vi "Create_Image_From_Pixmap_ARGB.vi"(8 "error in (no error)":errorcluster, 10 "Pixmap Image data":T1) -> (0 "error out":errorcluster, 3 "New ARGB Image":refnum<data-value>)   [LabVIEW 2020, in "g_ar_toolkit.lvlib"]
uses:
  g_ar_toolkit.lvlib
  <vilib>/picture/picture.llb/imagedata.ctl
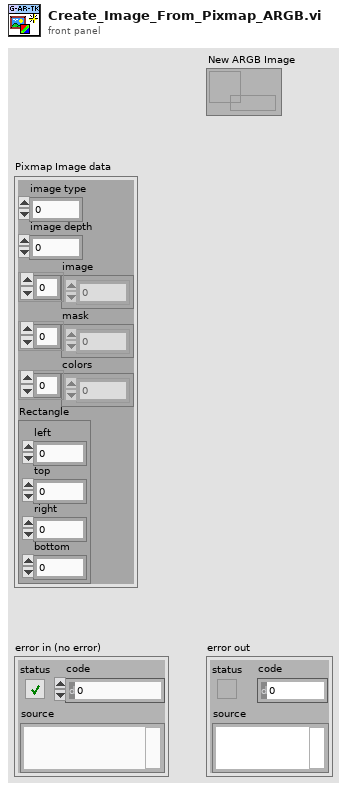
[diagram p1: front panel]
types:
  T1 = typedef "imagedata.ctl" = cluster{"image type":i32, "image depth":i32, "image":u8[], "mask":u8[], "colors":u32[], "Rectangle":cluster{"left":i16, "top":i16, "right":i16, "bottom":i16}}
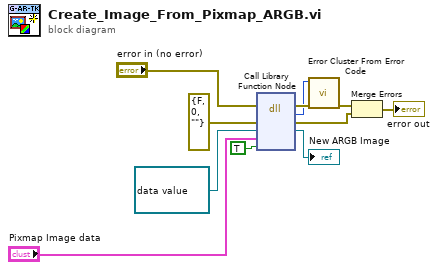
[diagram p0: block diagram]
diagram:
  n1 = dll-call lib="C:/serenial/libraries/g-augmented-reality-toolkit/LabVIEW/g_ar_toolkit/g_ar_toolkit.*.*" fn="Call Library Function Node"(error in="error in (no error)", "error_cluster"=errorcluster {"status"=FALSE, "code"=0, "source"=""} ("error constant"), "EDVR"=refnum<data-value> refnum, "ImageSize"="Pixmap Image data", "is_bgra"=TRUE) -> (error out=w7:errorcluster, "MgErr"=w6:i32, "error_cluster"=w1:errorcluster, "EDVR"=→"New ARGB Image":refnum<data-value>)  [unwired: 4 in, 1 out]
  n2 = call <vilib>:"Error Cluster From Error Code.vi"("error in (no error)"=w7, "error code (0)"=w6) -> ("error out"=w4:errorcluster)  [unwired: 7 in]
  n3 = Merge Errors(w4, w1) -> (→"error out":errorcluster)
